vi "checkLBValueNoEventClear.vi"() -> (0 "light barriers":bool[](array[boolean]))   [LabVIEW 2012]
uses:
  GlobalArduino.vi
  GlobalLB.vi
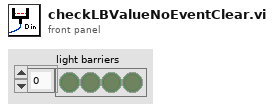
[diagram p1: front panel]
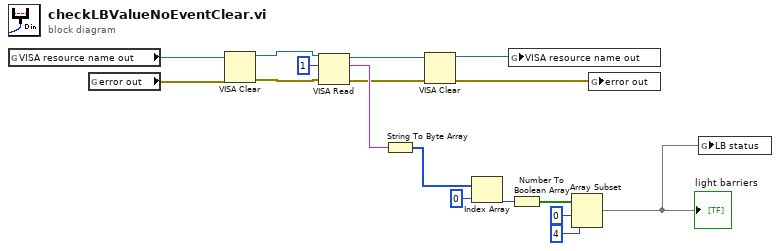
[diagram p0: block diagram]
diagram:
  n1 = global read "GlobalArduino.vi" "VISA resource name out"() -> (w4:refnum<visa-resource-name>)
  n2 = global read "GlobalArduino.vi" "error out"() -> (w2:errorcluster)
  n3 = VISA Clear(VISA resource name=w4, error in (no error)=w2) -> (VISA resource name out=w3:refnum<visa-resource-name>, error out=w1:errorcluster)
  n4 = VISA Read(VISA resource name=w3, byte count=u32 1, error in (no error)=w1) -> (VISA resource name out=w8:refnum<visa-resource-name>, read buffer=w16:string, error out=w6:errorcluster)  [unwired: 1 out]
  n5 = String To Byte Array(string=w16) -> (unsigned byte array=w15:u8[])
  n6 = VISA Clear(VISA resource name=w8, error in (no error)=w6) -> (VISA resource name out=w7:refnum<visa-resource-name>, error out=w5:errorcluster)
  n7 = Index Array(array=w15, index=0) -> (element=w13:u8)
  n8 = global write "GlobalArduino.vi" "VISA resource name out"(w7) -> ()
  n9 = Number To Boolean Array(number=w13) -> (Boolean array=w12:bool[])
  n10 = Array Subset(array=w12, index=0, length=4) -> (w9:bool[])
  "light barriers" <- w9
  n11 = global write "GlobalArduino.vi" "error out"(w5) -> ()
  n12 = global write "GlobalLB.vi" "LB status"(w9) -> ()
